vi "Run.vi"(8 "error in (no error)":errorcluster, 10 "TestCase":refnum<class "TestCase.lvclass">, 11 "TestResultMock in":refnum<class "TestResultMock.lvclass">) -> (0 "error out":errorcluster, 2 "TestCase out":refnum<class "TestCase.lvclass">, 3 "TestResultMock out":refnum<class "TestResultMock.lvclass">)   [LabVIEW 2019, in "TestCaseTestSupport.lvlib" / "TestResultMock.lvclass"]
doc: "Runs a <B>TestCase</B>."
uses:
  TestResultMock.lvclass
  TestCase/TestCase/TestCase.lvclass
  TestResultMock.lvclass/TestResultMock.ctl
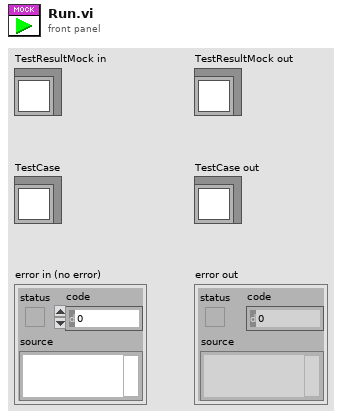
[diagram p1: front panel]
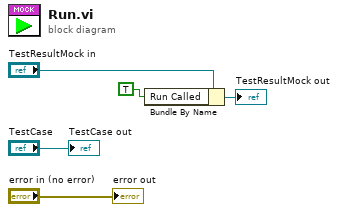
[diagram p0: block diagram]
diagram:
  n1 = Bundle By Name(cluster="TestResultMock in", "Run Called"=TRUE) -> (→"TestResultMock out":refnum<class "TestResultMock.lvclass">)
  "error out" <- "error in (no error)"
  "TestCase out" <- "TestCase"
